vi "_시리얼-패킷 데이타-수신.vi"(4 "ID":u8 format="%02x", 5 "전송 문자열":string="*IDN?", 6 "ErrIn":bool, 7 "시리얼 포트":refnum<visa-resource-name>="COM9") -> (0 "수신 문자열 버퍼":string, 1 "수신 문자열":string="LUMAXAERO,MEMS ADM,HW2.0,FW1.1", 2 "Processing TIme(ms)":u32=1, 3 "수신 실패(T)":bool)   [LabVIEW 2015]
panel:
  out "통신 재시도 횟수":i32
  out "통신 실패 횟수":u16
  out "웨이브폼 차트":u32(graph)=1
  out "에러 출력":errorcluster={"status"=FALSE, "code"=1073676294, "source"="_시리얼-패킷 데이타-수신.vi 안에 VISA 읽기"}
  out "수신 타이머 값":u32=5982350
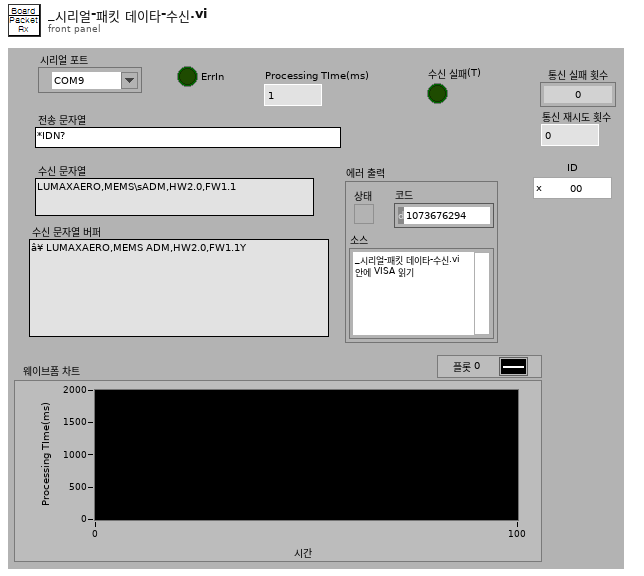
[diagram p1: front panel]
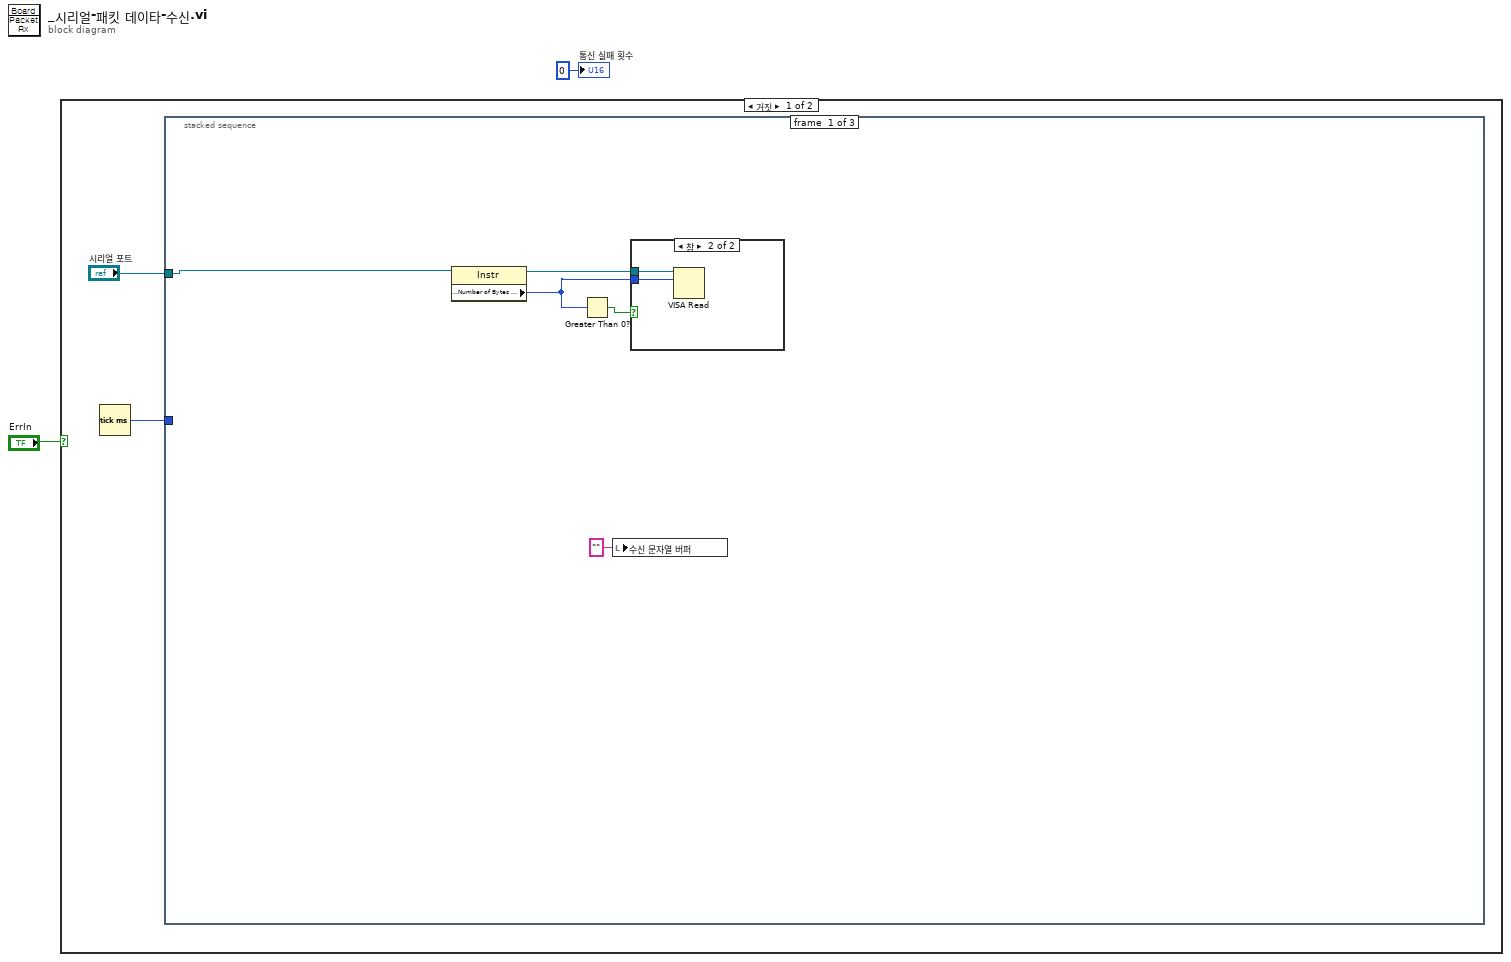
[diagram p0: block diagram]
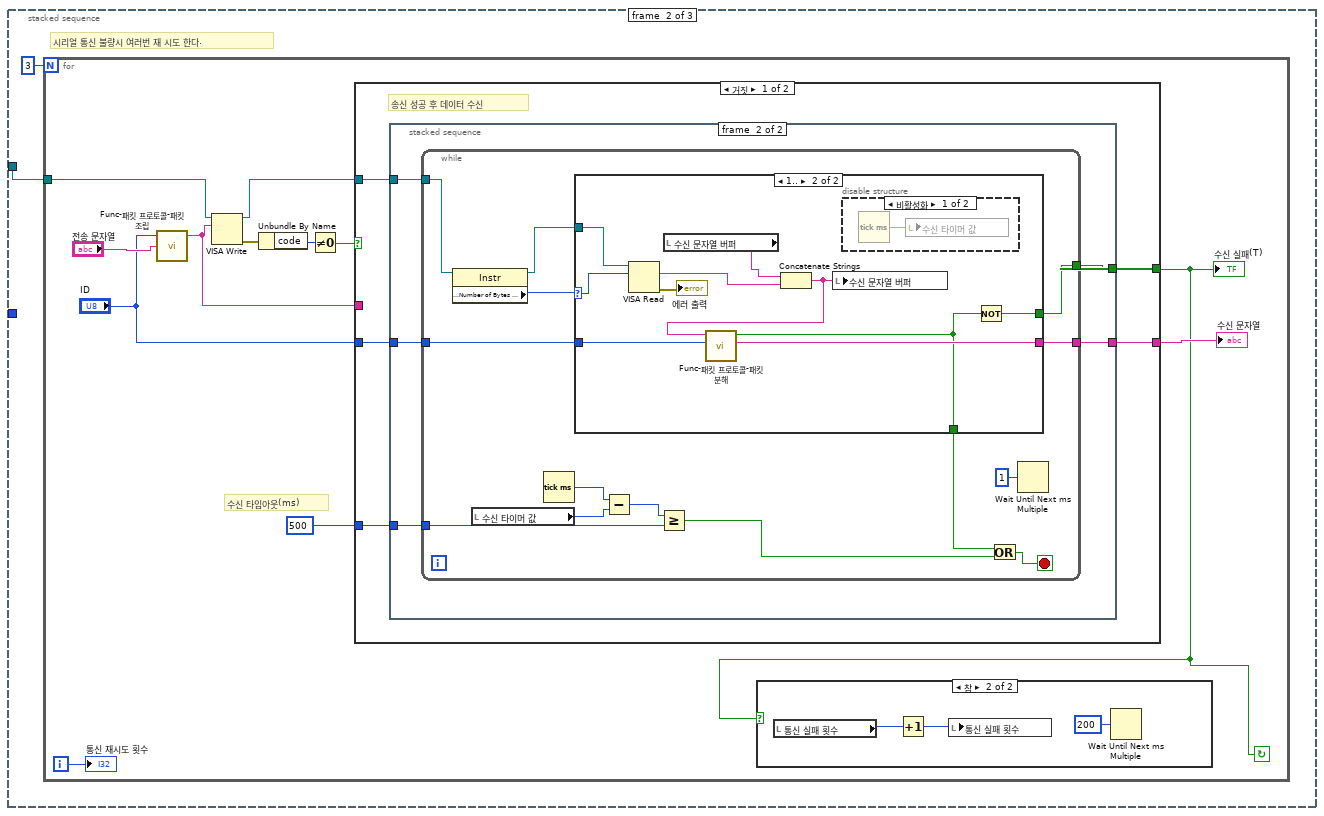
[diagram p3: hidden frame]
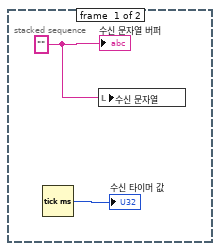
[diagram p5: hidden frame]
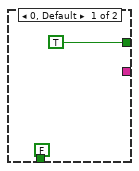
[diagram p6: hidden frame]
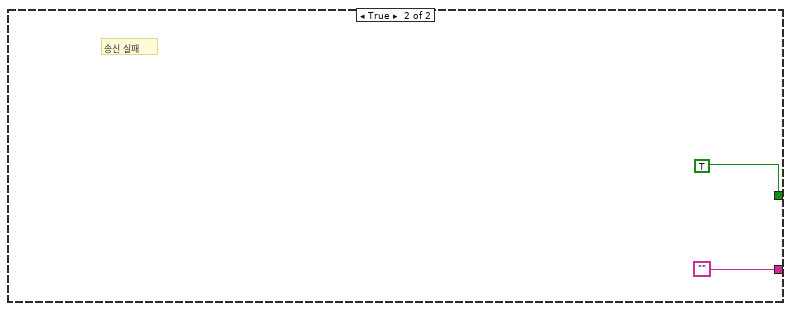
[diagram p8: hidden frame]
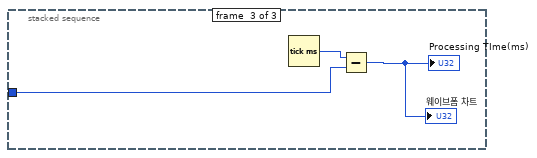
[diagram p9: hidden frame]
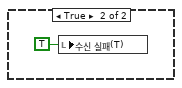
[diagram p10: hidden frame]
diagram:
  n1 = case shown="거짓" "ErrIn" {
    frame False {
      n2 = Tick Count (ms)() -> (millisecond timer value=w3:u32)
      n3 = stacked-sequence {
        tunnel: "시리얼 포트" -> [w8 w13 _]
        tunnel: w3 -> [_ _ w71]
        frame #0 {
          n4 = property class="Instr"(reference=w8) -> (reference out=w9:refnum<visa-resource-name>, "Serial Settings:Number of Bytes at Serial Port"=w6:u32)  [unwired: 1 in, 1 out]
          n5 = Greater Than 0?(x=w6) -> (x > 0?=w5:bool)
          n6 = local write "수신 문자열 버퍼"("" ("수신 문자열 버퍼")) -> ()
          n7 = case shown="참" w5 {
            tunnel: w9 -> [_ w11]
            tunnel: w6 -> [_ w10]
            frame False {
            }
            frame True {
              n8 = VISA Read(VISA resource name=w11, byte count=w10) -> ()  [unwired: 1 in, 4 out]
            }
          }
        }
        frame #1 {
          # "시리얼 통신 불량시 여러번 재 시도 한다."
          n9 = for {
            N: 3 -> [_]
            tunnel: w13 -> [w20]
            i -> [w17]
            stop <- w18 continue-if-true
            # "수신 타임아웃(ms)"
            n10 = call "Func-패킷 프로토콜-패킷 조립.vi"("메시지 데이터"="전송 문자열", "ID"="ID") -> ("패킷 데이터 (Hex)"=w14:string)  [unwired: 3 in]
            n11 = VISA Write(VISA resource name=w20, write buffer=w14) -> (VISA resource name out=w15:refnum<visa-resource-name>, error out=w25:errorcluster)  [unwired: 1 in, 1 out]
            n12 = Unbundle By Name(w25) -> ("code"=w24:i32)
            n13 = Not Equal To 0?(x=w24) -> (x != 0?=w23:bool)
            n14 = case shown="거짓" w23 {
              tunnel: [w30 ""] -> w21
              tunnel: [w31 TRUE] -> w18
              tunnel: w15 -> [w33 _]
              tunnel: 500 -> [w32 _]
              tunnel: "ID" -> [w29 _]
              tunnel: w14 -> [_ _]
              frame False {
                # "송신 성공 후 데이터 수신"
                n15 = stacked-sequence {
                  tunnel: w33 -> [_ w40]
                  tunnel: w32 -> [_ w39]
                  tunnel: [_ w37] -> w31
                  tunnel: [_ w38] -> w30
                  tunnel: w29 -> [_ w36]
                  frame #0 {
                    w34 = "" ("수신 문자열")
                    n16 = Tick Count (ms)() -> (millisecond timer value=→"수신 타이머 값":u32)
                    n17 = local write "수신 문자열"(w34) -> ()
                    "수신 문자열 버퍼" <- w34
                  }
                  frame #1 {
                    n18 = while {
                      tunnel: w40 -> [w54]
                      tunnel: w39 -> [w50]
                      tunnel: [w45] -> w38
                      tunnel: [w44] -> w37
                      tunnel: w36 -> [w42]
                      stop <- w49 stop-if-true
                      n19 = property class="Instr"(reference=w54) -> (reference out=w41:refnum<visa-resource-name>, "Serial Settings:Number of Bytes at Serial Port"=w47:u32)  [unwired: 1 in, 1 out]
                      n20 = local read "수신 타이머 값"() -> (w52:u32)
                      n21 = Tick Count (ms)() -> (millisecond timer value=w53:u32)
                      n22 = case shown="1.." w47 {
                        selector: w47 -> [_ w58]
                        tunnel: w41 -> [_ w65]
                        tunnel: [FALSE w60] -> w48
                        tunnel: [_ w61] -> w45
                        tunnel: [TRUE w59] -> w44
                        tunnel: w42 -> [_ w57]
                        frame 0, Default {
                        }
                        frame 1.. {
                          n23 = VISA Read(VISA resource name=w65, byte count=w58) -> (read buffer=w64:string, error out=→"에러 출력":errorcluster)  [unwired: 1 in, 2 out]
                          n24 = local read "수신 문자열 버퍼"() -> (w66:string)
                          n25 = Concatenate Strings(w66, w64) -> (w62:string)
                          n26 = call "Func-패킷 프로토콜-패킷 분해.vi"("ID"=w57, "메시지 데이터"=w62) -> ("메시지 데이터(Hex)"=w61:string, "패킷 정상"=w60:bool)  [unwired: 3 in, 1 out]
                          n27 = local write "수신 문자열 버퍼"(w62) -> ()
                          n28 = disable-structure shown="비활성화" {
                            frame Disabled {
                              n29 = Tick Count (ms)() -> (millisecond timer value=w67:u32)
                              n30 = local write "수신 타이머 값"(w67) -> ()
                            }
                            frame Enabled {
                            }
                          }
                          n31 = Not(x=w60) -> (.not. x?=w59:bool)
                        }
                      }
                      n32 = Subtract(x=w53, y=w52) -> (x-y=w51:u32)
                      n33 = Greater Or Equal?(x=w51, y=w50) -> (x >= y?=w46:bool)
                      n34 = Or(x=w48, y=w46) -> (x .or. y?=w49:bool)
                      n35 = Wait Until Next ms Multiple(millisecond multiple=u32 1 ("ms 배수")) -> ()  [unwired: 1 out]
                    }
                  }
                }
              }
              frame True {
                # "송신 실패"
              }
            }
            "수신 문자열" <- w21
            "수신 실패(T)" <- w18
            n36 = case shown="참" w18 {
              frame False {
              }
              frame True {
                n37 = local read "통신 실패 횟수"() -> (w27:u16)
                n38 = Increment(x=w27) -> (x+1=w26:u16)
                n39 = local write "통신 실패 횟수"(w26) -> ()
                n40 = Wait Until Next ms Multiple(millisecond multiple=u32 200 ("ms 배수")) -> ()  [unwired: 1 out]
              }
            }
            "통신 재시도 횟수" <- w17
          }
        }
        frame #2 {
          n41 = Tick Count (ms)() -> (millisecond timer value=w72:u32)
          n42 = Subtract(x=w72, y=w71) -> (x-y=→"Processing TIme(ms)" →"웨이브폼 차트":u32)
        }
      }
    }
    frame True {
      n43 = local write "수신 실패(T)"(TRUE ("수신 실패(T)")) -> ()
    }
  }
  "통신 실패 횟수" <- u16 0 ("통신 실패 횟수")
